vi "TAT_Start.vi"(8 "error In":errorcluster) -> (0 "error out":errorcluster)   [LabVIEW 2017]
uses:
  Controls/Ass. Loop Control.ctl
  <vilib>/Utility/error.llb/DialogType.ctl
panel:
  out "USER:-":string
  in  "Stop":bool
  out "DATE/TIME":string
  # "Nm"
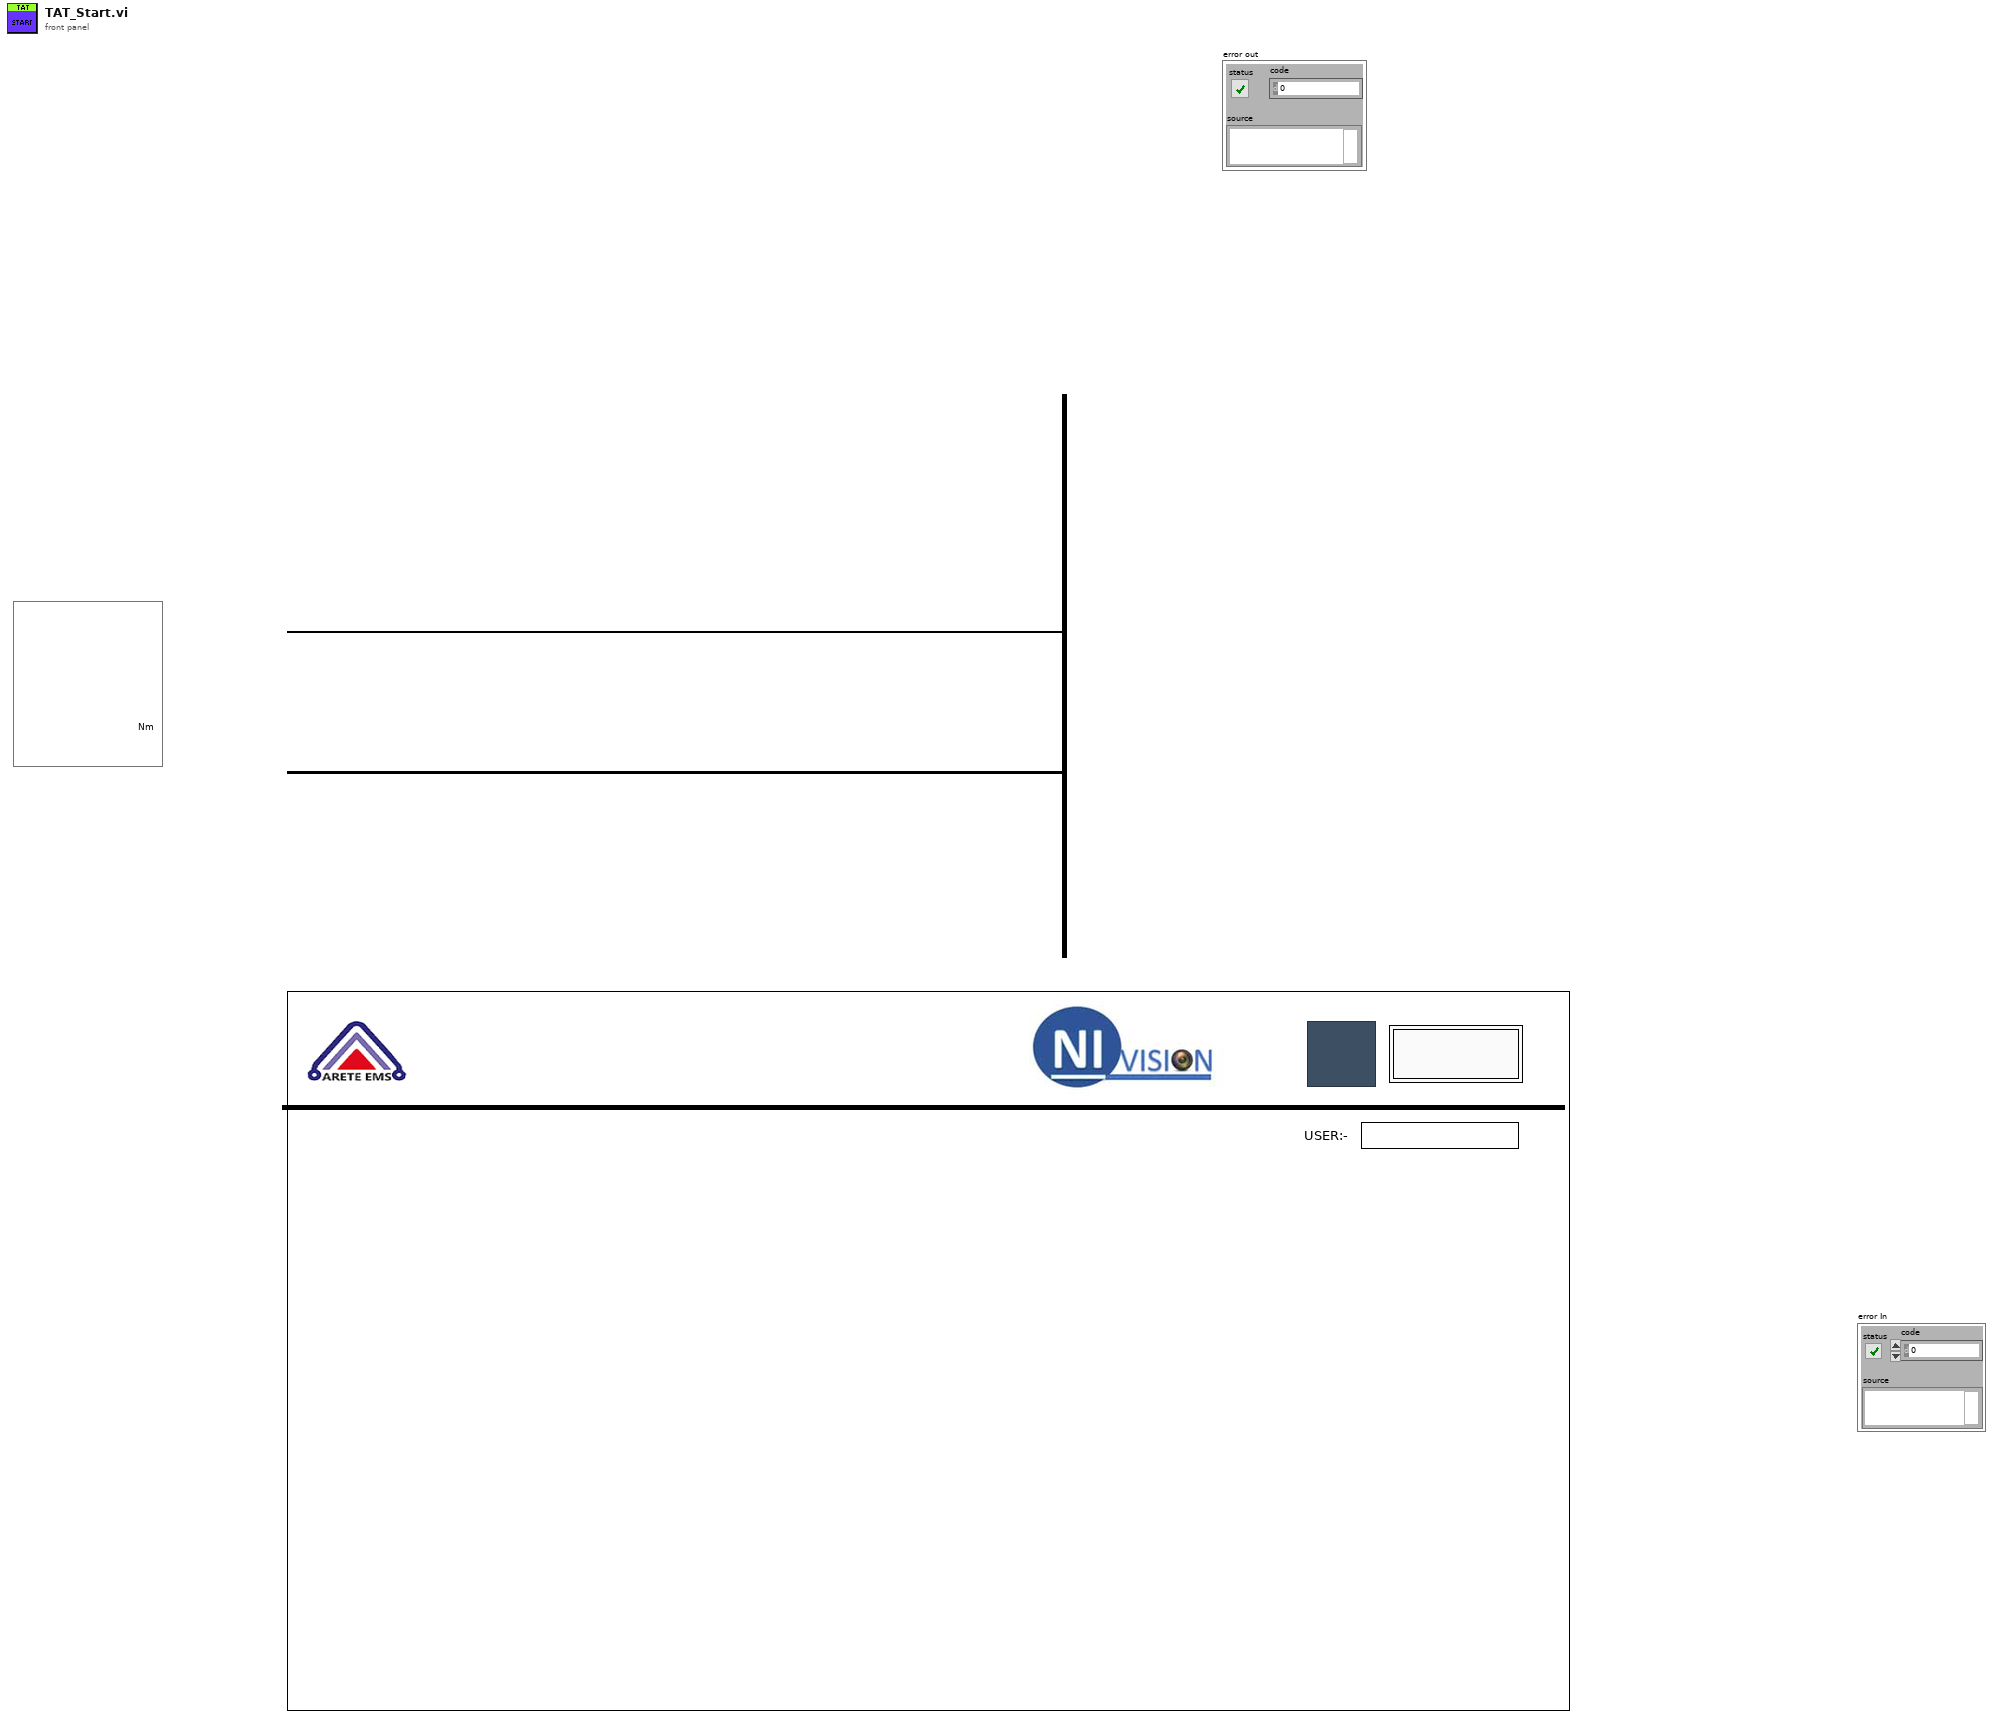
[diagram p1: front panel]
types:
  T1 = typedef "DialogType.ctl" = u16
  T2 = typedef "Ass. Loop Control.ctl" = enum16{"Package_Qty_Count", "GENERATE_QR_PRNT", "Cluster_update", "Waiting_for_scan", "barcode CHECK", "Int", "SaveReport ", "Barcode Print", "Start Cycle", "Wait", "Cycle End", "Stop"}
  T3 = enum32{"invalid app kind", "Development System", "Run Time System", "Student Edition", "Embedded LabVIEW", "Evaluation", "Custom"}
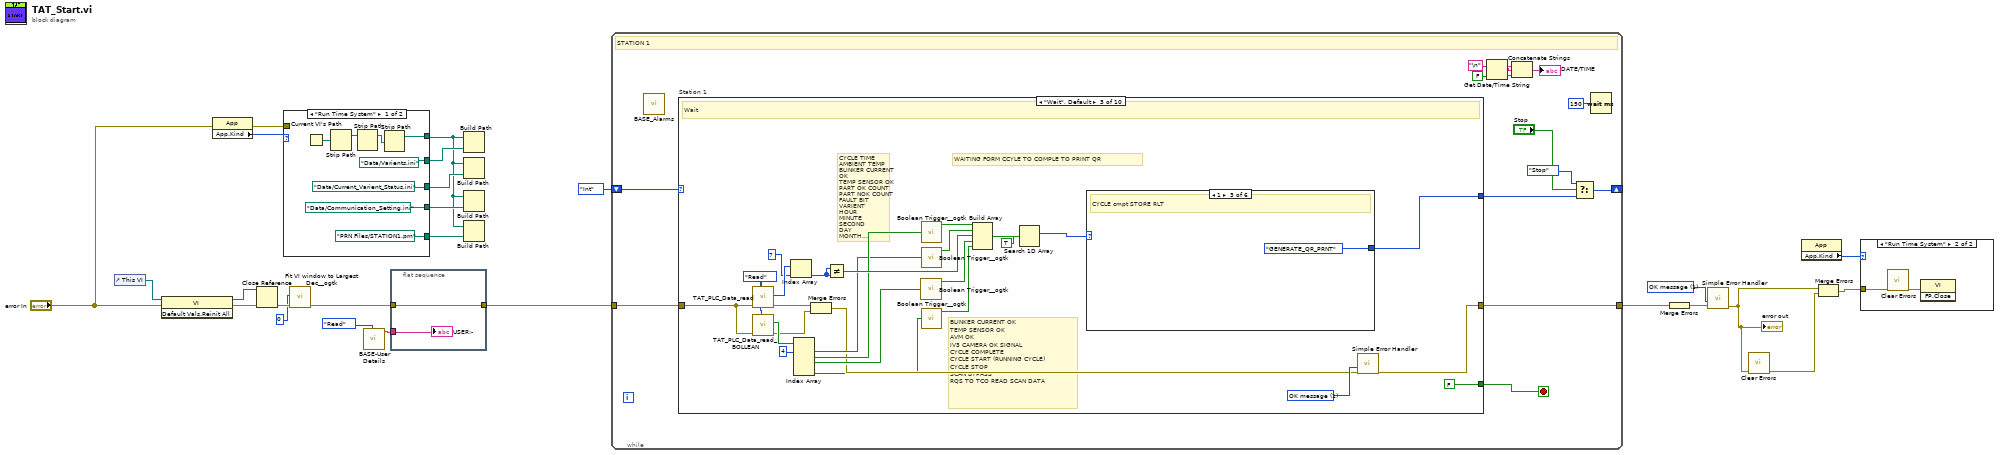
[diagram p0: block diagram]
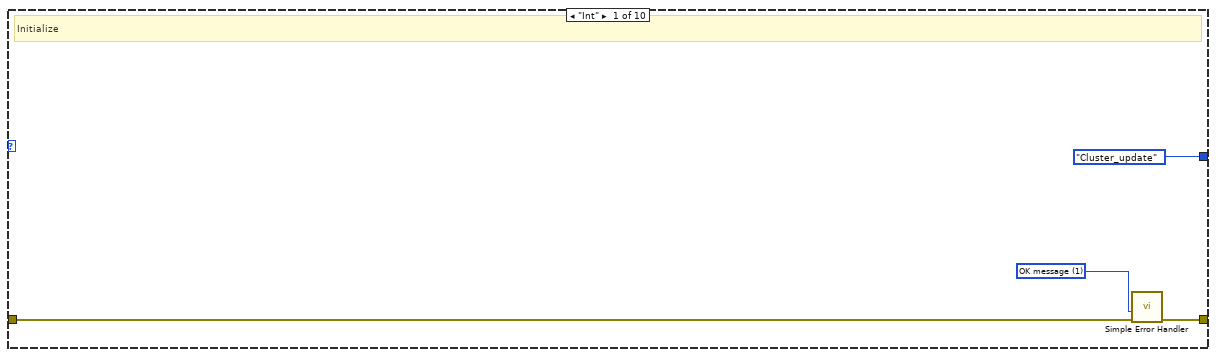
[diagram p3: hidden frame]
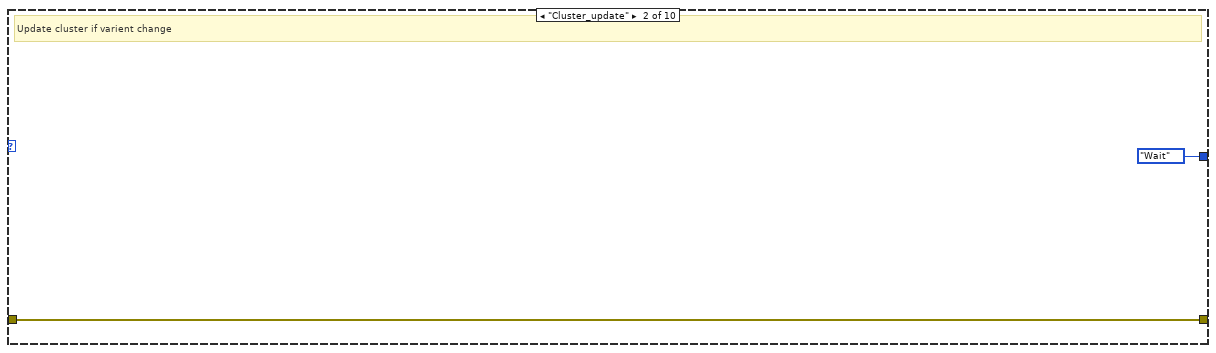
[diagram p4: hidden frame]
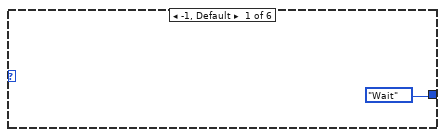
[diagram p5: hidden frame]
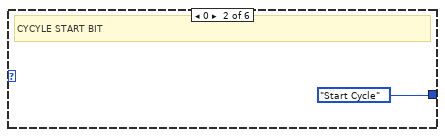
[diagram p6: hidden frame]
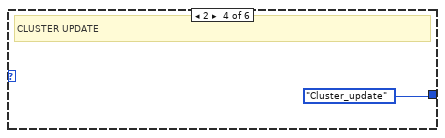
[diagram p7: hidden frame]
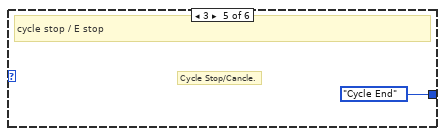
[diagram p8: hidden frame]
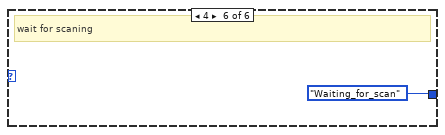
[diagram p9: hidden frame]
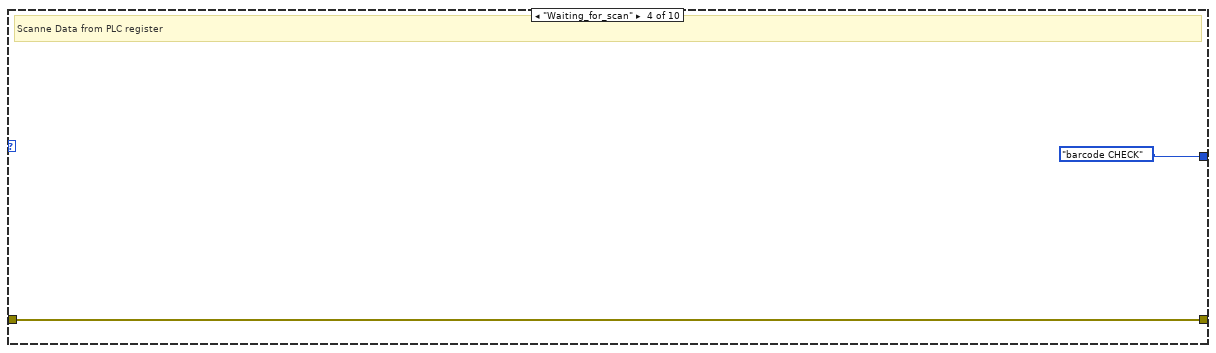
[diagram p10: hidden frame]
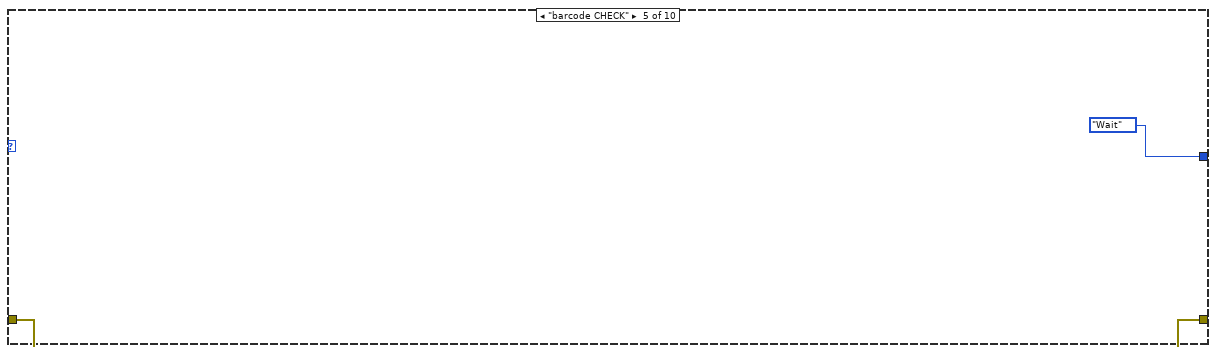
[diagram p11: hidden frame]
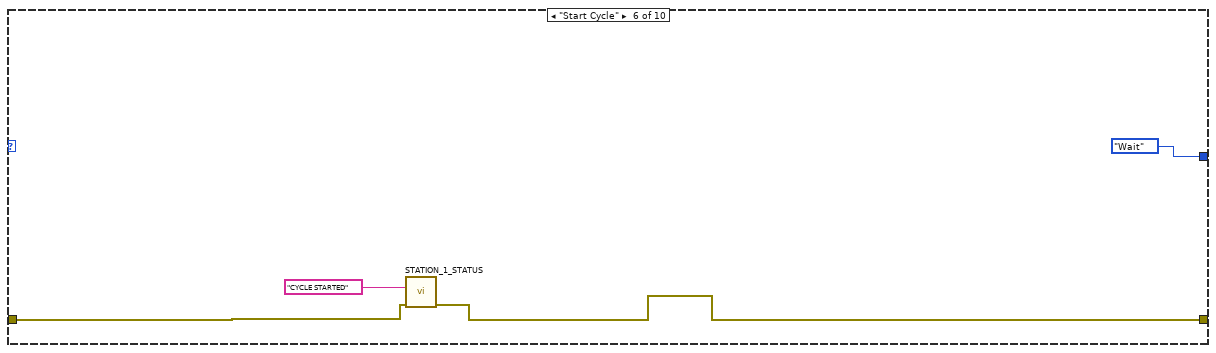
[diagram p12: hidden frame]
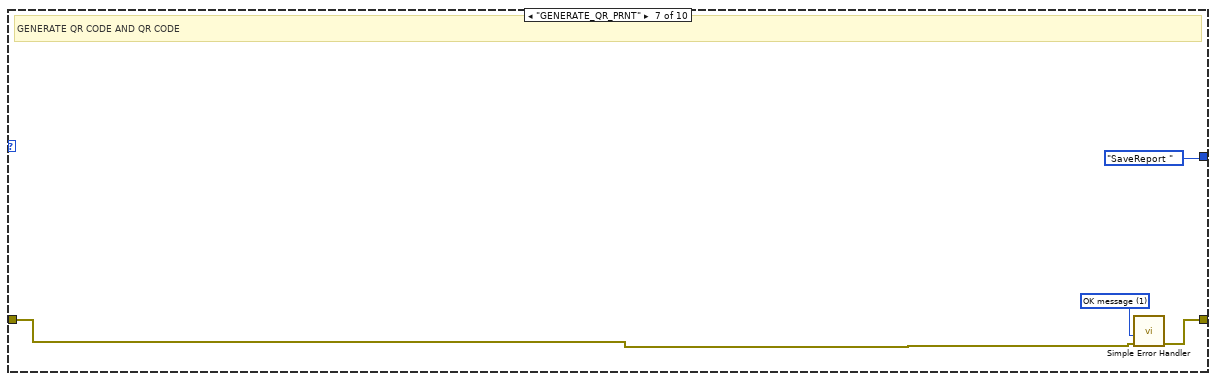
[diagram p13: hidden frame]
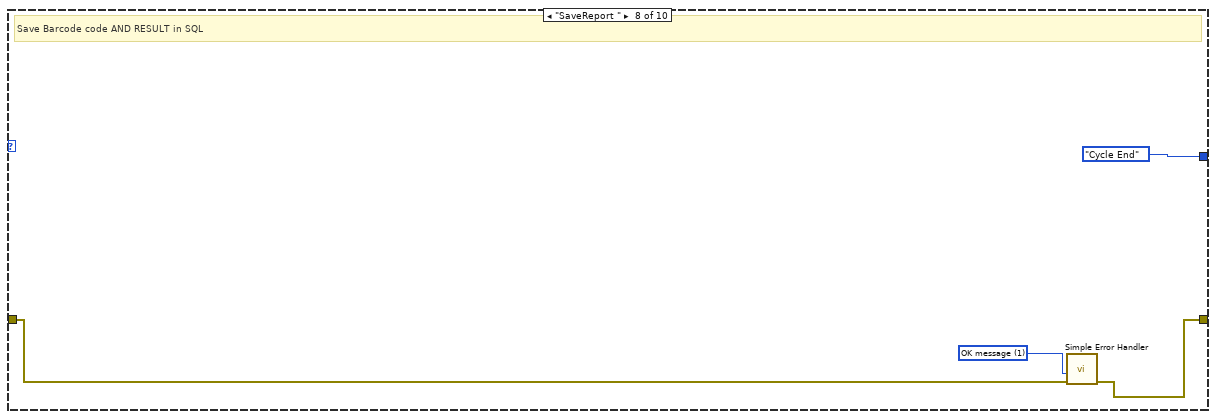
[diagram p14: hidden frame]
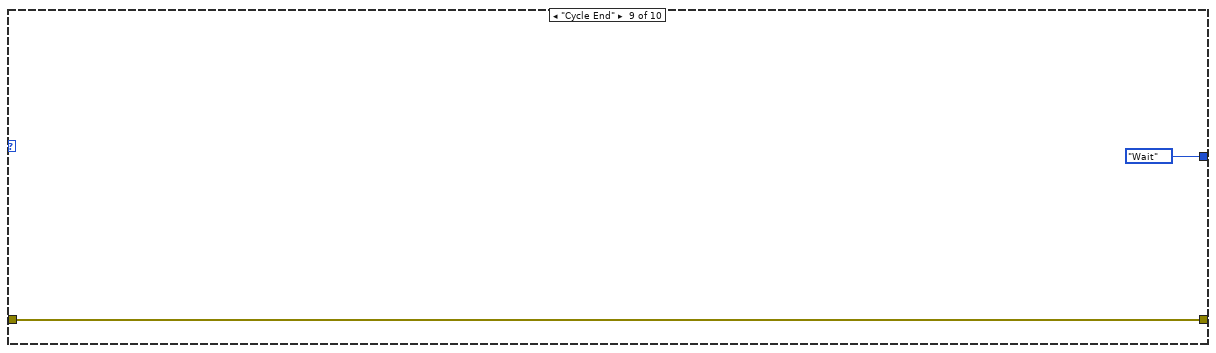
[diagram p15: hidden frame]
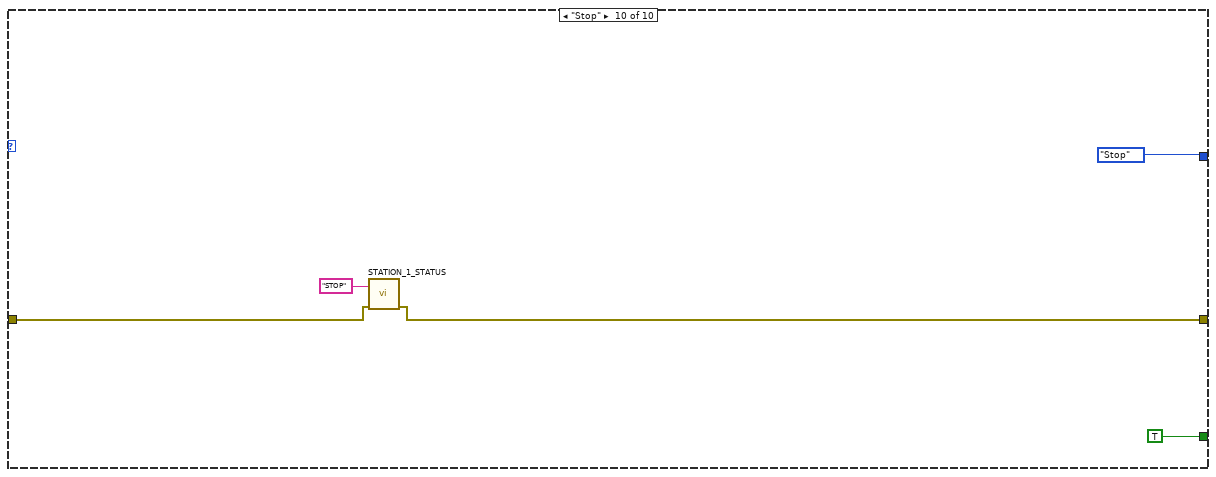
[diagram p16: hidden frame]
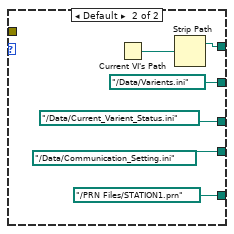
[diagram p17: hidden frame]
diagram:
  w16 = T1 1 items=["no dialog", "OK message", "continue or stop message", "OK message + warnings", "continue/stop + warnings"] ("type of dialog (OK msg:1)")
  n1 = control-ref of="This VI"() -> (w25:refnum<vi>)
  n2 = invoke class="VI" method="Default Vals.Reinit All"(reference=w25, error in="error In") -> (reference out=w23:refnum<vi>, error out=w24:errorcluster)  [unwired: 1 in, 1 out]
  n3 = property class="App"(error in="error In") -> (error out=w10:errorcluster, "App.Kind"=w14:T3)  [unwired: 1 in, 1 out]
  n4 = Close Reference(reference=w23, error in (no error)=w24) -> (error out=w22:errorcluster)
  n5 = case shown="\"Run Time System\"" w14 {
    tunnel: [path "Data/Varients.ini" ("path") path "../Data/Varients.ini" ("path")] -> w13
    tunnel: [w29 w37] -> w3
    tunnel: [path "Data/Current_Varient_Status.ini" ("path") path "../Data/Current_Varient_Status.ini" ("path")] -> w12
    tunnel: [path "Data/Communication_Setting.ini" ("path") path "../Data/Communication_Setting.ini" ("path")] -> w11
    tunnel: w10 -> [_ _]
    tunnel: [path "PRN Files/STATION1.prn" ("path") path "../PRN Files/STATION1.prn" ("path")] -> w8
    frame "Run Time System" {
      n6 = Current VI's Path() -> (path=w32:path)
      n7 = Strip Path(path=w32) -> (stripped path=w31:path)  [unwired: 1 out]
      n8 = Strip Path(path=w31) -> (stripped path=w30:path)  [unwired: 1 out]
      n9 = Strip Path(path=w30) -> (stripped path=w29:path)  [unwired: 1 out]
    }
    frame Default {
      n10 = Current VI's Path() -> (path=w38:path)
      n11 = Strip Path(path=w38) -> (stripped path=w37:path)  [unwired: 1 out]
    }
  }
  n12 = call <userlib>:"Fit VI window to Largest Dec__ogtk.vi"("error in (no error)"=w22, "border spacing (2 px)"=0) -> ("error out"=w7:errorcluster)  [unwired: 4 in, 1 out]
  n13 = call "BASE-User Details.vi"("Enum"=enum16{"Read", "Write"}."Read") -> ("User Name Out"=w17:string)  [unwired: 9 in, 1 out]
  n14 = flat-sequence {
    tunnel: [w41] -> w2
    tunnel: w7 -> [w41]
    tunnel: w17 -> [w40]
    frame #0 {
      "USER:-" <- w40
    }
  }
  n15 = Build Path(base path=w3, name or relative path=w13) -> ()  [unwired: 1 out]
  n16 = Build Path(base path=w3, name or relative path=w12) -> ()  [unwired: 1 out]
  n17 = Build Path(base path=w3, name or relative path=w11) -> ()  [unwired: 1 out]
  n18 = Build Path(base path=w3, name or relative path=w8) -> ()  [unwired: 1 out]
  n19 = while {
    tunnel: w2 -> [w42]
    shift-right: [w52] -> _
    shift-left: Ass._Loop_Control."Int" ("Enum") -> [w55]
    tunnel: [w53] -> w20
    stop <- w45 stop-if-true
    # "STATION 1"
    n20 = call "BASE_Alarms.vi"() -> ()  [unwired: 11 in, 1 out]
    n21 = case "Station 1" shown="\"Wait\", Default" w55 {
      tunnel: [Ass._Loop_Control."Cluster_update" ("Enum") Ass._Loop_Control."Wait" ("Enum") w81 Ass._Loop_Control."barcode CHECK" ("Enum") Ass._Loop_Control."Wait" ("Enum") Ass._Loop_Control."Wait" ("Enum") Ass._Loop_Control."SaveReport " ("Enum") Ass._Loop_Control."Cycle End" ("Enum") Ass._Loop_Control."Wait" ("Enum") Ass._Loop_Control."Stop" ("Enum")] -> w44
      tunnel: [_ _ FALSE _ _ _ _ _ _ TRUE] -> w45
      tunnel: [w57 w60 w78 w94 w96 w98 w104 w107 w110 w112] -> w53
      tunnel: w42 -> [w56 w60 w75 w94 w96 w99 w102 w106 w110 w113]
      frame "Int" {
        w58 = T1 1 items=["no dialog", "OK message", "continue or stop message", "OK message + warnings", "continue/stop + warnings"] ("type of dialog (OK msg:1)")
        # "Initialize"
        n22 = call <vilib>:"Simple Error Handler.vi"("type of dialog (OK msg:1)"=w58, "error in (no error)"=w56) -> ("error out"=w57:errorcluster)  [unwired: 3 in, 4 out]
      }
      frame "Cluster_update" {
        # "Update cluster if varient change"
      }
      frame "Wait", Default {
        w79 = T1 1 items=["no dialog", "OK message", "continue or stop message", "OK message + warnings", "continue/stop + warnings"] ("type of dialog (OK msg:1)")
        w76 = enum16{"Read", "Write"}."Read" ("Enum")
        # "CYCLE TIME\nAMBIENT TEMP\nBLINKER CURRENT OK\nTEMP SENSOR OK\nPART OK COUNT\nPART NOK COUNT\nFAULT BIT\nVARIENT\nHOUR\nMINUTE\nSECOND\nDAY\nMONTH\nYEAR\nSERIAL NUMBER"
        # "BLINKER CURRENT OK\nTEMP SENSOR OK\nAVM OK\nIV3 CAMERA OK SIGNAL\nCYCLE COMPLETE\nCYCLE START (RUNNING CYCLE)\nCYCLE STOP\nSCAN BYPASS\nRQS TO TCO READ SCAN DATA"
        # "WAITING FORM CCYLE TO COMPLE TO PRINT QR"
        # "Wait"
        n23 = call "TAT_PLC_Data_read.vi"("Enum"=w76, "error in (no error)"=w75) -> ("error out"=w66:errorcluster, "Array 2"=w82:u16[])  [unwired: 8 in]
        n24 = call "TAT_PLC_Data_read_BOLLEAN.vi"("Enum"=w76, "error in (no error)"=w75) -> ("error out"=w64:errorcluster, "Array 2"=w74:bool[])  [unwired: 8 in]
        n25 = Index Array(array=w82, index=7) -> (element=w62:u16)
        n26 = Index Array(array=w74, index #1=4 ("index")) -> (element #1=w71:bool, element #2=w72:bool, element #3=w70:bool, element #5=w63:bool)  [unwired: 4 in, 1 out]
        n27 = Merge Errors(w66, w64) -> (w65:errorcluster)
        n28 = Not Equal?(x=w62, y=w62) -> (x != y?=w80:bool)
        n29 = call <userlib>:"Boolean Trigger__ogtk.vi"("Boolean Input"=w70) -> ("Rising Edge"=w69:bool)  [unwired: 1 in, 1 out]
        n30 = call <userlib>:"Boolean Trigger__ogtk.vi"("Boolean Input"=w72) -> ("Rising Edge"=w86:bool)  [unwired: 1 in, 1 out]
        n31 = call <userlib>:"Boolean Trigger__ogtk.vi"("Boolean Input"=w71) -> ("Rising Edge"=w77:bool)  [unwired: 1 in, 1 out]
        n32 = call <userlib>:"Boolean Trigger__ogtk.vi"("Boolean Input"=w63) -> ("Rising Edge"=w68:bool)  [unwired: 1 in, 1 out]
        n33 = Build Array(w86, w77, w80, w69, w68) -> (w85:bool[])
        n34 = Search 1D Array(1D array=w85, element=TRUE ("Boolean Input")) -> (index of element=w84:i32)  [unwired: 1 in]
        n35 = case shown="1" w84 {
          tunnel: [Ass._Loop_Control."Wait" ("Enum") Ass._Loop_Control."Start Cycle" ("Enum") Ass._Loop_Control."GENERATE_QR_PRNT" ("Enum") Ass._Loop_Control."Cluster_update" ("Enum") Ass._Loop_Control."Cycle End" ("Enum") Ass._Loop_Control."Waiting_for_scan" ("Enum")] -> w81
          frame -1, Default {
          }
          frame 0 {
            # "CYCYLE START BIT"
          }
          frame 1 {
            # "CYCLE cmpt STORE RLT"
          }
          frame 2 {
            # "CLUSTER UPDATE"
          }
          frame 3 {
            # "Cycle Stop/Cancle."
            # "cycle stop / E stop"
          }
          frame 4 {
            # "wait for scaning"
          }
        }
        n36 = call <vilib>:"Simple Error Handler.vi"("type of dialog (OK msg:1)"=w79, "error in (no error)"=w65) -> ("error out"=w78:errorcluster)  [unwired: 3 in, 4 out]
      }
      frame "Waiting_for_scan" {
        # "Scanne Data from PLC register"
      }
      frame "barcode CHECK" {
      }
      frame "Start Cycle" {
        n37 = call "STATION_1_STATUS.vi"("error in (no error)"=w99, "STATUS"="CYCLE STARTED" ("Cycle Status")) -> ("error out"=w98:errorcluster)  [unwired: 9 in]
      }
      frame "GENERATE_QR_PRNT" {
        w105 = T1 1 items=["no dialog", "OK message", "continue or stop message", "OK message + warnings", "continue/stop + warnings"] ("type of dialog (OK msg:1)")
        # "GENERATE QR CODE AND QR CODE"
        n38 = call <vilib>:"Simple Error Handler.vi"("type of dialog (OK msg:1)"=w105, "error in (no error)"=w102) -> ("error out"=w104:errorcluster)  [unwired: 3 in, 4 out]
      }
      frame "SaveReport " {
        w108 = T1 1 items=["no dialog", "OK message", "continue or stop message", "OK message + warnings", "continue/stop + warnings"] ("type of dialog (OK msg:1)")
        # "Save Barcode code AND RESULT in SQL"
        n39 = call <vilib>:"Simple Error Handler.vi"("type of dialog (OK msg:1)"=w108, "error in (no error)"=w106) -> ("error out"=w107:errorcluster)  [unwired: 3 in, 4 out]
      }
      frame "Cycle End" {
      }
      frame "Stop" {
        n40 = call "STATION_1_STATUS.vi"("error in (no error)"=w113, "STATUS"="STOP" ("Cycle Status")) -> ("error out"=w112:errorcluster)  [unwired: 9 in]
      }
    }
    n41 = Get Date/Time String(want seconds? (F)=FALSE) -> (date string=w49:string, time string=w48:string)  [unwired: 2 in]
    n42 = Concatenate Strings(w49, "\n", w48) -> (→"DATE/TIME":string)
    n43 = Select(t=Ass._Loop_Control."Stop" ("Enum"), s="Stop", f=w44) -> (s? t:f=w52:T2)
    n44 = Wait (ms)(milliseconds to wait=u32 150) -> ()  [unwired: 1 out]
  }
  n45 = Merge Errors(w20) -> (w19:errorcluster)
  n46 = call <vilib>:"Simple Error Handler.vi"("type of dialog (OK msg:1)"=w16, "error in (no error)"=w19) -> ("error out"=w4:errorcluster)  [unwired: 3 in, 4 out]
  "error out" <- w4
  n47 = call <vilib>:"Clear Errors.vi"("error in (no error)"=w4) -> ("error out"=w1:errorcluster)  [unwired: 5 in, 1 out]
  n48 = property class="App"() -> ("App.Kind"=w15:T3)  [unwired: 2 in, 2 out]
  n49 = Merge Errors(w4, w1) -> (w5:errorcluster)
  n50 = case shown="\"Run Time System\"" w15 {
    tunnel: w5 -> [_ w118]
    frame "invalid app kind", Default {
    }
    frame "Run Time System" {
      n51 = call <vilib>:"Clear Errors.vi"("error in (no error)"=w118) -> ("error out"=w117:errorcluster)  [unwired: 5 in, 1 out]
      n52 = invoke class="VI" method="FP.Close"(error in=w117) -> ()  [unwired: 2 in, 3 out]
    }
  }
